vi "thcd_400_qt.vi"(7 "stop_external":refnum<vi>) -> ()   [LabVIEW 2019]
uses:
  thcd_controls/ctrl_chn_thcd.ctl
  thcd_controls/ctrl_sms_thcd.ctl
  <vilib>/Analysis/baseanly.llb/Mean (DBL).vi
  thcd_commands/thcd_set_samp.vi
  thcd_commands/thcd_get_samp.vi
  <vilib>/Analysis/NI_AALBase.lvlib
panel:
  in  "n_avg":i32=10
  out "current_point_ch1":dbl caption="Current S.P."
  in  "close":bool
  in  "open":bool
  out "status_log":bool caption="Status"
  in  "Logging":bool=TRUE
  out "Last Updated":timestamp format="%<%Y-%m-%d %H:%M:%S>T"
  out "Sensor data":cluster{cluster{"X":dbl, "Y":dbl}[]}[](graph)
  out "thcd_st":bool caption="Status"
  out "thcd_res_msg":string caption="Msg"
  in  "thcd_val":dbl=0.1 caption="Set Point" min=0.1 max=10000.0 format="%#_5f"
  in  "wait_sec":u32=5 caption="Interval (s)"
  out "thcd_res_4":T2
  out "thcd_res_3":T2
  out "thcd_res_2":T2
  out "thcd_res_1":T2
  in  "getstat":bool
  in  "set":bool
  in  "read":bool
  out "FC1":dbl caption="L/m" format="%.2f"
  in  "Baud_rate":u32(ring)=9600 items=["9.6KHz"=9600, "19.2KHz"=19200]
  in  "VISA":refnum<visa-resource-name>="COM37"
  in  "Init Devices":bool
  in  "Exit":bool
  # "Do Not Close This"
  # "THCD-400 for QT"
  # "Flow Control: FC1 (Ch 1)"
  # "QT FCB:"
  # "\"res_state\" must be \"CLOSE\" (which actually means \"AUTO\") to control the flow rates remotely.  If it is not, change it by using the hardware button of THCD-400."
  # "Set Range:\n0.1-10000"
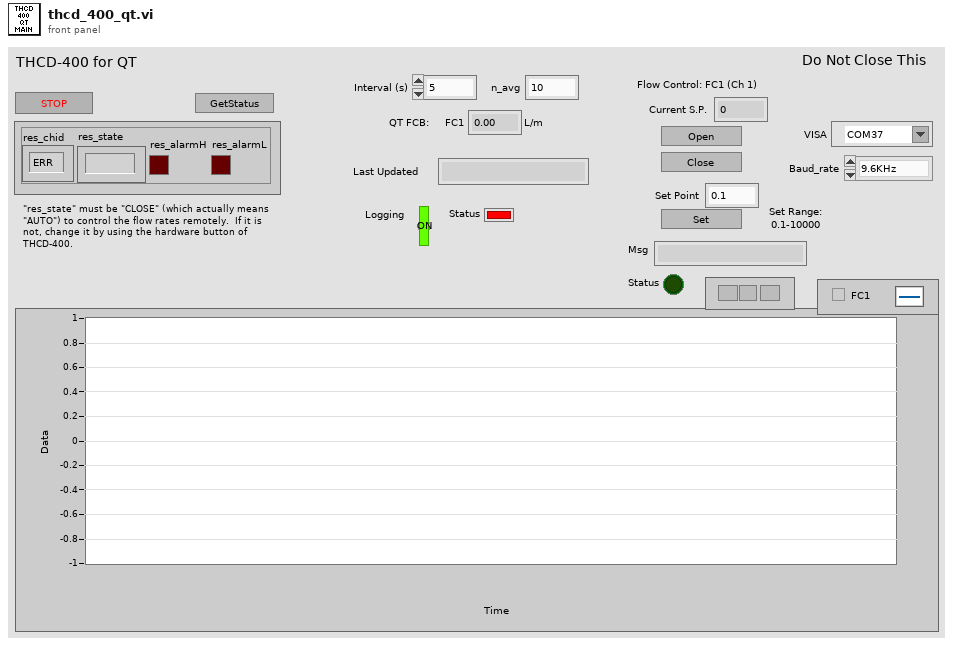
[diagram p1: front panel]
types:
  T1 = typedef "ctrl_chn_thcd.ctl" = enum8{"ERR", "1", "2", "3", "4"}
  T2 = cluster{"res_chid":T1, "res_state":string, "res_alarmH":bool, "res_alarmL":bool}
  T3 = typedef "ctrl_sms_thcd.ctl" = enum16{"idle", "init", "exit", "read", "enable_auto_ctrl_ch1", "enable_auto_ctrl_ch2", "open", "close", "mode_ch1", "set", "open_ch2", "close_ch2", "mode_ch2", "set_ch2", "getstat"}
  T4 = enum16{"SetPoint", "AlarmH", "AlarmL", "Multiplier", "CalibValue"}
  T5 = cluster{"res_chid":T1, "res_val":dbl, "res_uom":string, "res_gid":string}[]
  T6 = cluster{"res_chid":T1, "res_val":dbl, "res_uom":string, "res_gid":string}
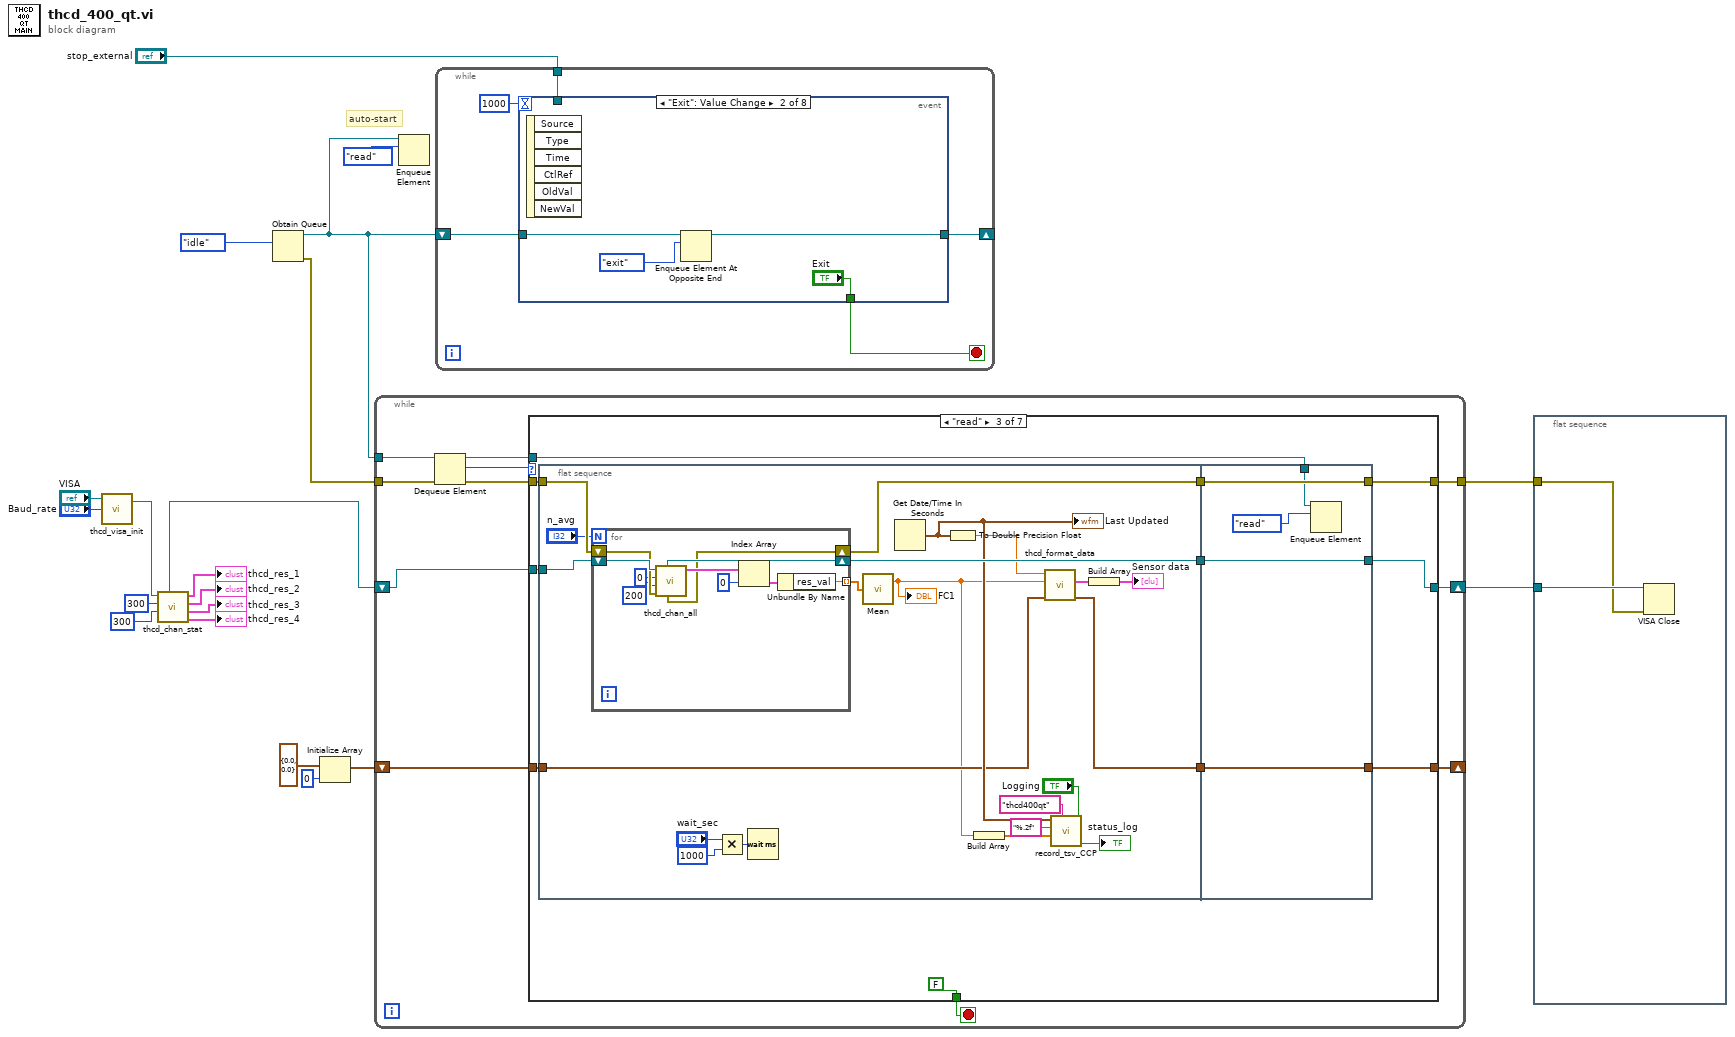
[diagram p0: block diagram]
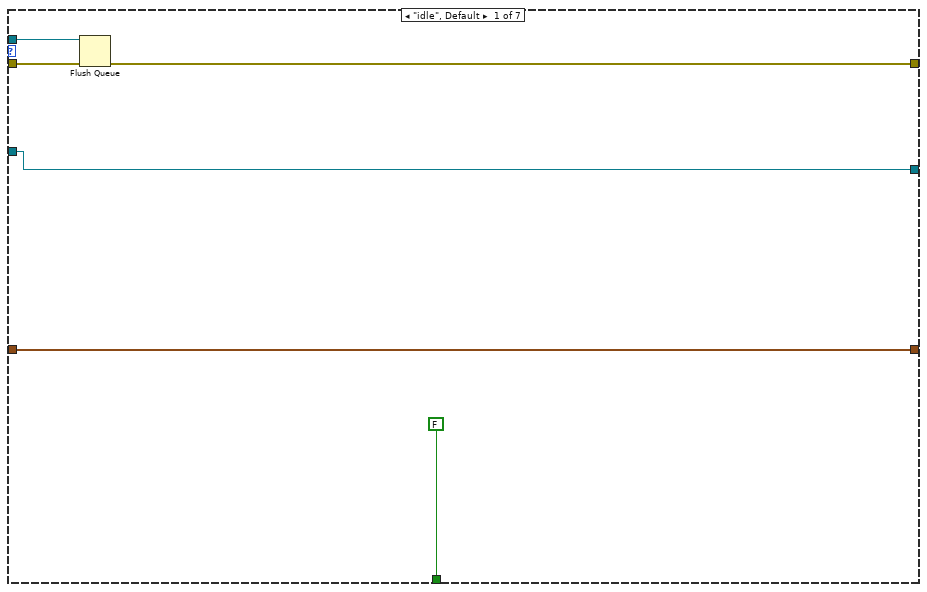
[diagram p2: hidden frame]
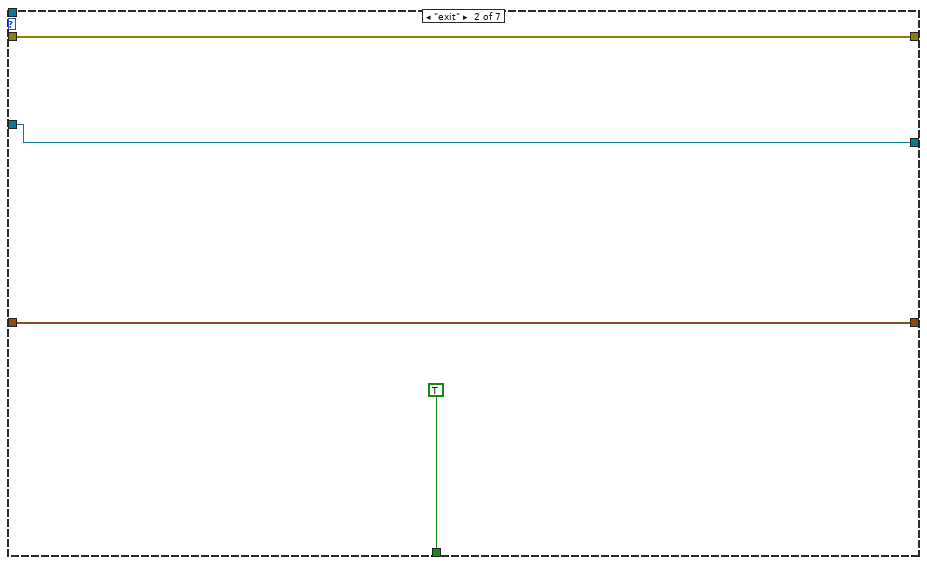
[diagram p3: hidden frame]
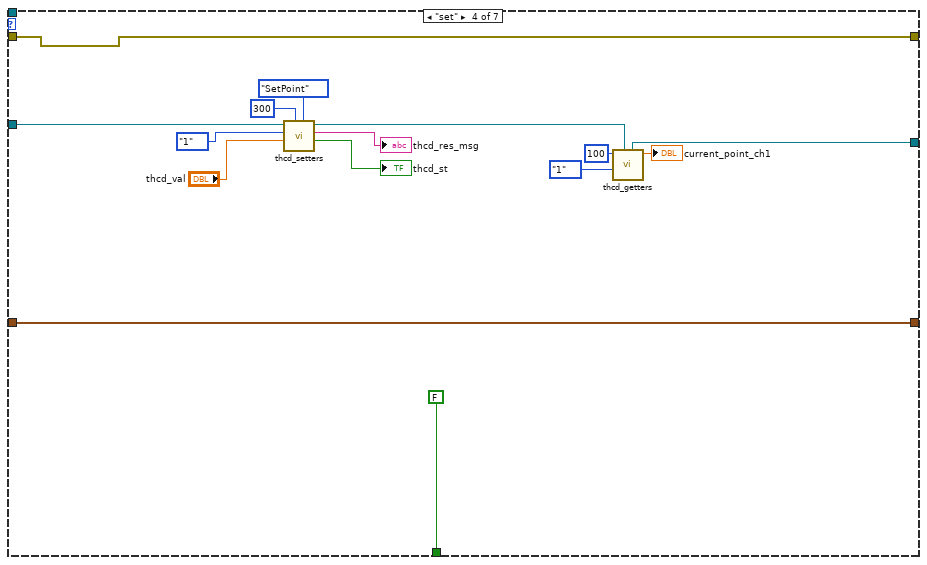
[diagram p4: hidden frame]
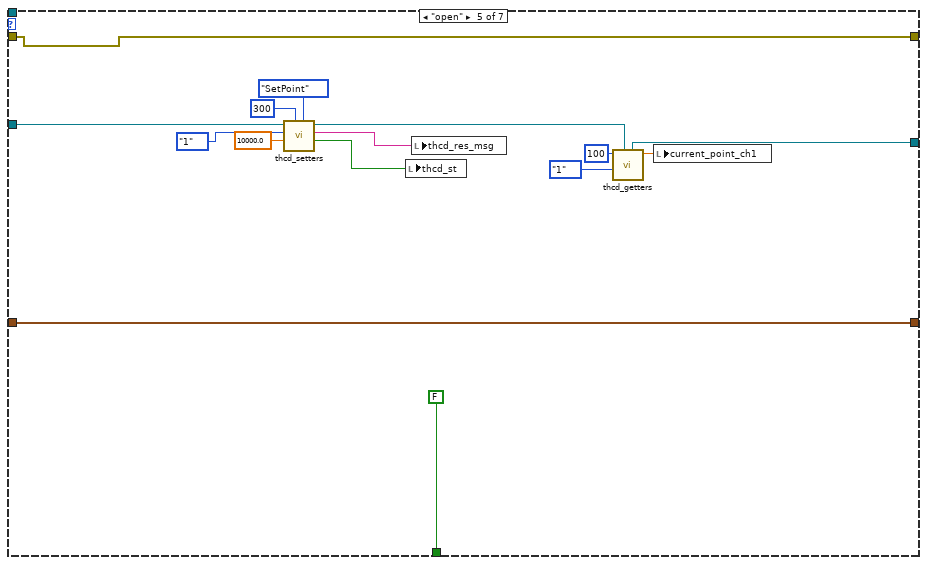
[diagram p5: hidden frame]
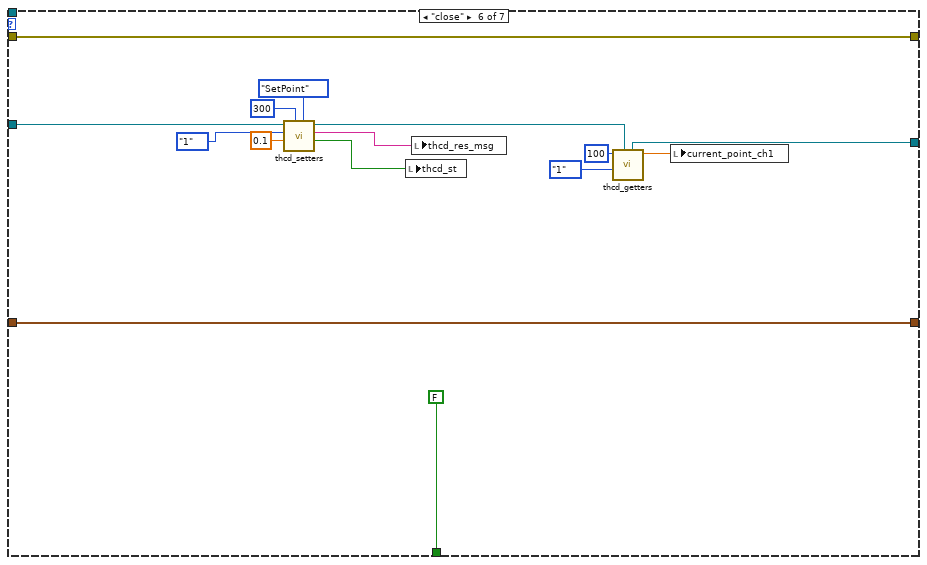
[diagram p6: hidden frame]
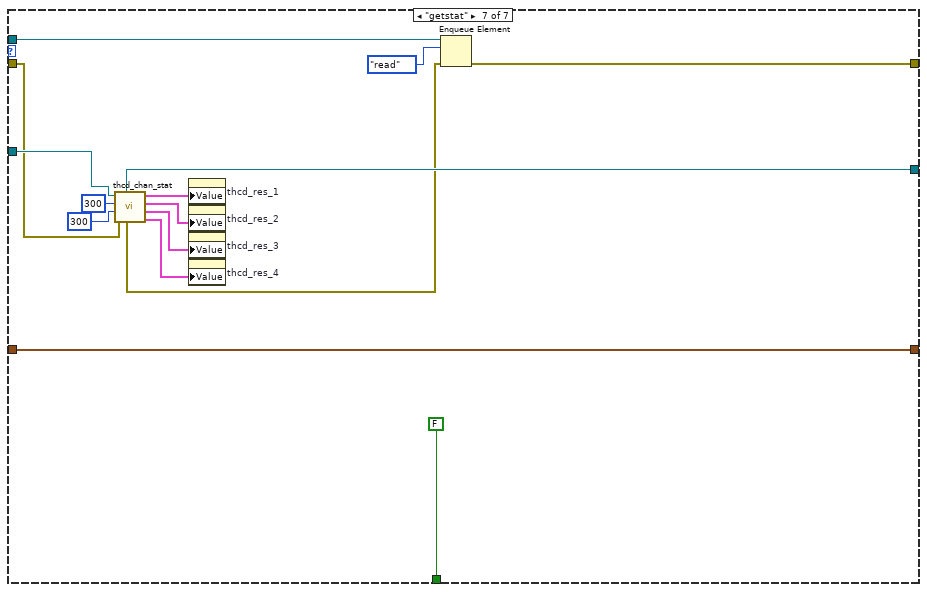
[diagram p7: hidden frame]
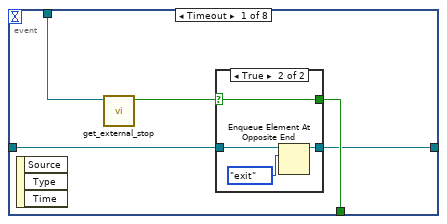
[diagram p8: hidden frame]
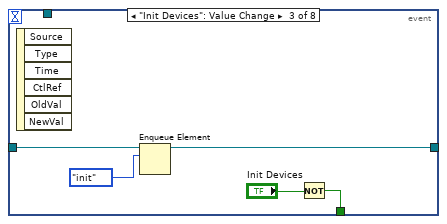
[diagram p10: hidden frame]
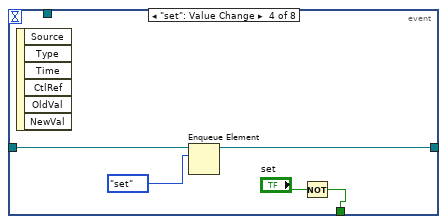
[diagram p11: hidden frame]
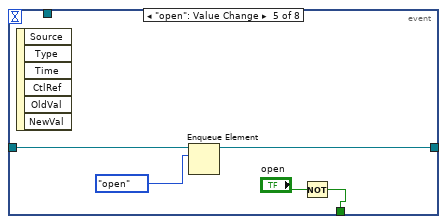
[diagram p12: hidden frame]
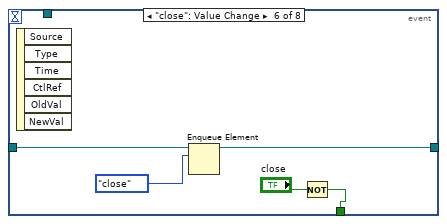
[diagram p13: hidden frame]
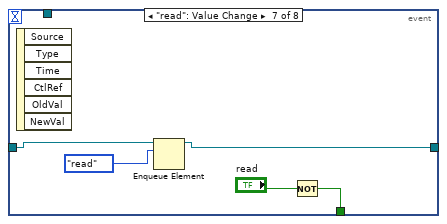
[diagram p14: hidden frame]
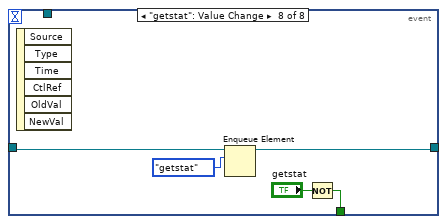
[diagram p15: hidden frame]
diagram:
  # "auto-start"
  n1 = call "thcd_visa_init.vi"("Serial Settings:Baud Rate"="Baud_rate", "thcd_visa"="VISA") -> ("thcd_visa"=w7:refnum<visa-resource-name>)  [unwired: 1 in, 1 out]
  n2 = call "thcd_chan_stat.vi"("thcd_b2r"=u32 300, "thcd_delay"=u32 300, "thcd_visa"=w7) -> ("thcd_res_4"=→"thcd_res_4":T2, "thcd_res_3"=→"thcd_res_3":T2, "thcd_res_2"=→"thcd_res_2":T2, "thcd_res_1"=→"thcd_res_1":T2, "thcd_visa"=w6:refnum<visa-resource-name>)  [unwired: 1 in, 3 out]
  n3 = Obtain Queue(element data type=ctrl_sms_thcd."idle" ("Enum")) -> (queue out=w4:refnum<queue>, error out=w19:errorcluster)  [unwired: 4 in, 1 out]
  n4 = Initialize Array(cluster{"X":dbl, "Y":dbl} {"X"=0.0, "Y"=0.0}, 0 ("dimension size")) -> (w16:cluster{"X":dbl, "Y":dbl}[])
  n5 = while {
    tunnel: w19 -> [w29]
    tunnel: [w26] -> w2
    tunnel: w4 -> [w30]
    shift-right: [w21] -> w3
    shift-left: w6 -> [w24]
    shift-right: [w22] -> _
    shift-left: w16 -> [w23]
    stop <- w31 stop-if-true
    n6 = Dequeue Element(queue=w30, error in (no error)=w29) -> (queue out=w25:refnum<queue>, element=w28:T3, error out=w27:errorcluster)  [unwired: 1 in, 1 out]
    n7 = case shown="\"read\"" w28 {
      tunnel: w25 -> [w36 _ w42 _ _ _ w147]
      tunnel: [FALSE TRUE FALSE FALSE FALSE FALSE FALSE] -> w31
      tunnel: w27 -> [w35 w40 w51 w102 w104 w132 w135]
      tunnel: [w34 w40 w49 w102 w104 w132 w146] -> w26
      tunnel: [w33 w39 w50 w92 w106 w120 w140] -> w21
      tunnel: w24 -> [w33 w39 w52 w101 w117 w131 w141]
      tunnel: w23 -> [w32 w38 w47 w94 w113 w127 w144]
      tunnel: [w32 w38 w46 w94 w113 w127 w144] -> w22
      frame "idle", Default {
        n8 = Flush Queue(queue=w36, error in (no error)=w35) -> (error out=w34:errorcluster)  [unwired: 2 out]
      }
      frame "exit" {
      }
      frame "read" {
        n9 = flat-sequence {
          tunnel: w52 -> [w73]
          tunnel: w51 -> [w72]
          tunnel: w47 -> [w63]
          tunnel: [w71] -> w45
          tunnel: [w70] -> w44
          tunnel: [w62] -> w43
          tunnel: [w86] -> w46
          tunnel: [w87] -> w49
          tunnel: [w88] -> w50
          tunnel: w45 -> [w88]
          tunnel: w44 -> [w87]
          tunnel: w43 -> [w86]
          tunnel: w42 -> [w85]
          frame #0 {
            n10 = for {
              N: "n_avg" -> [_]
              tunnel: [w74] -> w58 mode=indexing
              shift-right: [w79] -> w71
              shift-left: w73 -> [w83]
              shift-right: [w75] -> w70
              shift-left: w72 -> [w82]
              n11 = call "thcd_chan_all.vi"("err_in"=w82, "thcd_b2r"=u32 200, "thcd_delay"=u32 0, "thcd_visa"=w83) -> ("thcd_res"=w76:T5, "err_out"=w75:errorcluster, "thcd_visa"=w79:refnum<visa-resource-name>)  [unwired: 3 in, 2 out]
              n12 = Index Array(array=w76, index=0) -> (element=w77:T6)
              n13 = Unbundle By Name(w77) -> ("res_val"=w74:dbl)
            }
            n14 = Multiply(x="wait_sec", y=u32 1000) -> (x*y=w56:u32)
            n15 = Wait (ms)(milliseconds to wait=w56) -> ()  [unwired: 1 out]
            n16 = call-poly <vilib>:"Mean.vi"("X"=w58) -> ("mean"=w57:dbl)  [unwired: 1 out]
            "FC1" <- w57
            n17 = Get Date/Time In Seconds() -> (seconds since 1Jan1904=w65:timestamp)
            "Last Updated" <- w65
            n18 = To Double Precision Float(number=w65) -> (double precision float=w60:dbl)
            n19 = Build Array(w57) -> (w64:dbl[])
            n20 = call "thcd_format_data.vi"("array_in"=w63, "value"=w57, "time"=w60) -> ("array_out"=w62:cluster{"time":dbl, "value":dbl}[], "cluster_out"=w61:cluster{cluster{"time":dbl, "value":dbl}[]})  [unwired: 7 in]
            n21 = call "record_tsv_CCP.vi"("logging_on"="Logging", "folder_name"="thcd400qt", "value_array"=w64, "format"="%.2f", "time"=w65) -> ("status"=→"status_log":bool)  [unwired: 5 in, 1 out]
            n22 = Build Array(w61) -> (→"Sensor data":cluster{cluster{"time":dbl, "value":dbl}[]}[])
          }
          frame #1 {
            n23 = Enqueue Element(queue=w85, element=ctrl_sms_thcd."read") -> ()  [unwired: 2 in, 3 out]
          }
        }
      }
      frame "set" {
        n24 = call-poly "thcd_setters.vi"("thcd_com"=T4."SetPoint", "thcd_delay"=u32 300, "thcd_val"="thcd_val", "thcd_ch"=ctrl_chn_thcd."1", "thcd_visa"=w101) -> ("thcd_st"=→"thcd_st":bool, "thcd_res_msg"=→"thcd_res_msg":string, "thcd_visa"=w93:refnum<visa-resource-name>)  [unwired: 1 in, 1 out]
        n25 = call-poly "thcd_getters.vi"("thcd_visa"=w93, "thcd_ch"=ctrl_chn_thcd."1", "thcd_delay"=u32 100) -> ("thcd_res"=→"current_point_ch1":dbl, "thcd_visa"=w92:refnum<visa-resource-name>)  [unwired: 3 in, 4 out]
      }
      frame "open" {
        n26 = call-poly "thcd_setters.vi"("thcd_com"=T4."SetPoint", "thcd_delay"=u32 300, "thcd_val"=10000.0, "thcd_ch"=ctrl_chn_thcd."1", "thcd_visa"=w117) -> ("thcd_st"=w110:bool, "thcd_res_msg"=w111:string, "thcd_visa"=w107:refnum<visa-resource-name>)  [unwired: 1 in, 1 out]
        n27 = local write "thcd_st"(w110) -> ()
        n28 = local write "thcd_res_msg"(w111) -> ()
        n29 = call-poly "thcd_getters.vi"("thcd_visa"=w107, "thcd_ch"=ctrl_chn_thcd."1", "thcd_delay"=u32 100) -> ("thcd_res"=w105:dbl, "thcd_visa"=w106:refnum<visa-resource-name>)  [unwired: 3 in, 4 out]
        n30 = local write "current_point_ch1"(w105) -> ()
      }
      frame "close" {
        n31 = call-poly "thcd_setters.vi"("thcd_com"=T4."SetPoint", "thcd_delay"=u32 300, "thcd_val"=0.1, "thcd_ch"=ctrl_chn_thcd."1", "thcd_visa"=w131) -> ("thcd_st"=w124:bool, "thcd_res_msg"=w125:string, "thcd_visa"=w121:refnum<visa-resource-name>)  [unwired: 1 in, 1 out]
        n32 = local write "thcd_st"(w124) -> ()
        n33 = local write "thcd_res_msg"(w125) -> ()
        n34 = call-poly "thcd_getters.vi"("thcd_visa"=w121, "thcd_ch"=ctrl_chn_thcd."1", "thcd_delay"=u32 100) -> ("thcd_res"=w119:dbl, "thcd_visa"=w120:refnum<visa-resource-name>)  [unwired: 3 in, 4 out]
        n35 = local write "current_point_ch1"(w119) -> ()
      }
      frame "getstat" {
        n36 = call "thcd_chan_stat.vi"("err_in"=w135, "thcd_b2r"=u32 300, "thcd_delay"=u32 300, "thcd_visa"=w141) -> ("thcd_res_4"=w136:T2, "thcd_res_3"=w137:T2, "thcd_res_2"=w138:T2, "thcd_res_1"=w139:T2, "err_out"=w134:errorcluster, "thcd_visa"=w140:refnum<visa-resource-name>)  [unwired: 2 out]
        n37 = property on="thcd_res_1" class="Clust (strict)"("Value"=w139) -> ()  [unwired: 2 in, 2 out]
        n38 = property on="thcd_res_2" class="Clust (strict)"("Value"=w138) -> ()  [unwired: 2 in, 2 out]
        n39 = property on="thcd_res_3" class="Clust (strict)"("Value"=w137) -> ()  [unwired: 2 in, 2 out]
        n40 = property on="thcd_res_4" class="Clust (strict)"("Value"=w136) -> ()  [unwired: 2 in, 2 out]
        n41 = Enqueue Element(queue=w147, element=ctrl_sms_thcd."read", error in (no error)=w134) -> (error out=w146:errorcluster)  [unwired: 1 in, 2 out]
      }
    }
  }
  n42 = Enqueue Element(queue=w4, element=ctrl_sms_thcd."read") -> ()  [unwired: 2 in, 3 out]
  n43 = while {
    shift-right: [w152] -> _
    shift-left: w4 -> [w153]
    tunnel: "stop_external" -> [w150]
    stop <- w151 stop-if-true
    n44 = event shown="[1] \"Exit\": Value Change" {
      selector: _ -> [_ _ _ _ _ _ _ _]
      dyn-events: _ -> [_ _ _ _ _ _ _ _]
      timeout: 1000 -> [_ _ _ _ _ _ _ _]
      tunnel: w153 -> [w157 w168 w173 w175 w180 w185 w191 w196]
      tunnel: [w156 w167 w172 w174 w179 w184 w190 w195] -> w152
      tunnel: [w158 "Exit" w169 w177 w182 w187 w192 w197] -> w151
      tunnel: w150 -> [w155 _ _ _ _ _ _ _]
      event Timeout {
        n45 = event-data() -> ()  [unwired: 1 in, 3 out]
        n46 = call "get_external_stop.vi"("ref_stop_external"=w155) -> ("stop_output"=w154:bool)  [unwired: 10 in]
        n47 = case shown="True" w154 {
          selector: w154 -> [w160 w164]
          tunnel: [w160 w164] -> w158
          tunnel: w157 -> [w159 w161]
          tunnel: [w159 w162] -> w156
          frame False {
          }
          frame True {
            n48 = Enqueue Element At Opposite End(queue=w161, element=ctrl_sms_thcd."exit" ("Enum")) -> (queue out=w162:refnum<queue>)  [unwired: 2 in, 2 out]
          }
        }
      }
      event "Exit": Value Change {
        n49 = event-data() -> ()  [unwired: 1 in, 6 out]
        n50 = Enqueue Element At Opposite End(queue=w168, element=ctrl_sms_thcd."exit" ("Enum")) -> (queue out=w167:refnum<queue>)  [unwired: 2 in, 2 out]
      }
      event "Init Devices": Value Change {
        n51 = event-data() -> ()  [unwired: 1 in, 6 out]
        n52 = Enqueue Element(queue=w173, element=ctrl_sms_thcd."init") -> (queue out=w172:refnum<queue>)  [unwired: 2 in, 2 out]
        n53 = Not(x="Init Devices") -> (.not. x?=w169:bool)
      }
      event "set": Value Change {
        n54 = event-data() -> ()  [unwired: 1 in, 6 out]
        n55 = Enqueue Element(queue=w175, element=ctrl_sms_thcd."set" ("Enum")) -> (queue out=w174:refnum<queue>)  [unwired: 2 in, 2 out]
        n56 = Not(x="set") -> (.not. x?=w177:bool)
      }
      event "open": Value Change {
        n57 = event-data() -> ()  [unwired: 1 in, 6 out]
        n58 = Enqueue Element(queue=w180, element=ctrl_sms_thcd."open" ("Enum")) -> (queue out=w179:refnum<queue>)  [unwired: 2 in, 2 out]
        n59 = Not(x="open") -> (.not. x?=w182:bool)
      }
      event "close": Value Change {
        n60 = event-data() -> ()  [unwired: 1 in, 6 out]
        n61 = Enqueue Element(queue=w185, element=ctrl_sms_thcd."close" ("Enum")) -> (queue out=w184:refnum<queue>)  [unwired: 2 in, 2 out]
        n62 = Not(x="close") -> (.not. x?=w187:bool)
      }
      event "read": Value Change {
        n63 = event-data() -> ()  [unwired: 1 in, 6 out]
        n64 = Enqueue Element(queue=w191, element=ctrl_sms_thcd."read" ("Enum")) -> (queue out=w190:refnum<queue>)  [unwired: 2 in, 2 out]
        n65 = Not(x="read") -> (.not. x?=w192:bool)
      }
      event "getstat": Value Change {
        n66 = event-data() -> ()  [unwired: 1 in, 6 out]
        n67 = Enqueue Element(queue=w196, element=ctrl_sms_thcd."getstat") -> (queue out=w195:refnum<queue>)  [unwired: 2 in, 2 out]
        n68 = Not(x="getstat") -> (.not. x?=w197:bool)
      }
    }
  }
  n69 = flat-sequence {
    tunnel: w3 -> [w200]
    tunnel: w2 -> [w199]
    frame #0 {
      n70 = VISA Close(VISA resource name=w200, error in (no error)=w199) -> ()  [unwired: 1 out]
    }
  }
